vi "FTW-Actor-Initialized.vi"(0 "FTW Actor Instance":refnum<class "FTW-ActorExtended.lvclass">, 5 "Initialized Response":string, 11 "error in":errorcluster) -> (4 "FTW Actor Instance out":refnum<class "FTW-ActorExtended.lvclass">, 15 "error out":errorcluster)   [LabVIEW 2015, in "FTW-ActorExtended.lvclass"]
uses:
  FTW-ActorExtended.lvclass
  FTW-ActorExtended.lvclass/FTW-ActorExtended.ctl
  Instance/FTW-ActorInstance.lvclass
panel:
  out "Initialized Response String":string
  # "Inputs"
  # "Outputs"
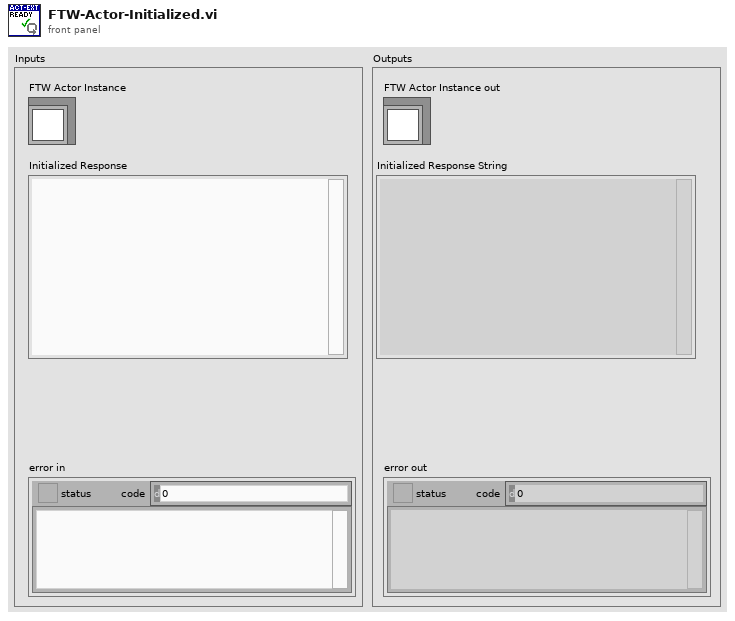
[diagram p1: front panel]
types:
  T1 = typedef "FTW-Type-JSON.ctl" = refnum<data-value>
  T2 = cluster{"Name":string, "URI":string, "Publisher":refnum<class "FTW-Publisher.lvclass">}[]
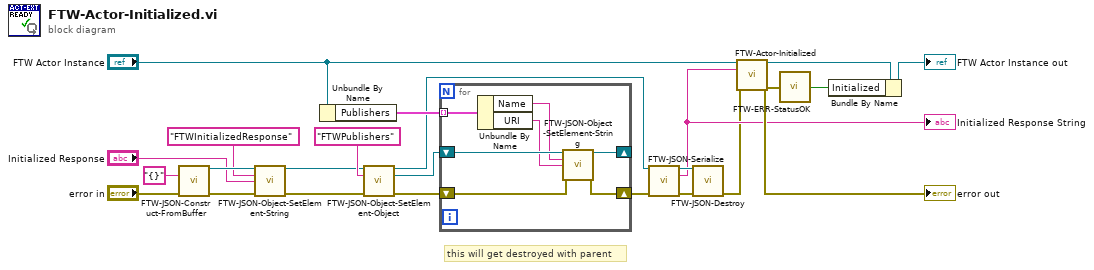
[diagram p0: block diagram]
diagram:
  # "this will get destroyed with parent"
  n1 = call "FTW-JSON-Construct-FromBuffer.vi"("JSON String (UTF-8)"="{}", "error in"="error in") -> ("JSON"=w16:T1, "error out"=w17:errorcluster)  [unwired: 12 in]
  n2 = call "FTW-JSON-Object-SetElement-String.vi"("JSON"=w16, "Key"="FTWInitializedResponse", "Value"="Initialized Response", "error in"=w17) -> ("JSON out"=w3:T1, "error out"=w4:errorcluster)  [unwired: 10 in]
  n3 = Unbundle By Name("FTW Actor Instance") -> ("Publishers"=w12:T2)
  n4 = call "FTW-JSON-Object-SetElement-Object.vi"("JSON Object"=w3, "Key"="FTWPublishers", "error in"=w4) -> ("JSON Root Object"=w7:T1, "JSON Sub-Object"=w10:T1, "error out"=w11:errorcluster)  [unwired: 10 in]
  n5 = for {
    shift-right: [w30] -> w2
    shift-left: w11 -> [w24]
    tunnel: w12 -> [w27] mode=indexing
    shift-right: [w28] -> _
    shift-left: w10 -> [w29]
    n6 = Unbundle By Name(w27) -> ("Name"=w26:string, "URI"=w25:string)
    n7 = call "FTW-JSON-Object-SetElement-String.vi"("JSON"=w29, "Key"=w26, "Value"=w25, "error in"=w24) -> ("JSON out"=w28:T1, "error out"=w30:errorcluster)  [unwired: 10 in]
  }
  n8 = call "FTW-JSON-Serialize.vi"("JSON"=w7, "error in"=w2) -> ("JSON out"=w6:T1, "JSON String (UTF-8)"=w5:string, "error out"=w8:errorcluster)  [unwired: 11 in]
  "Initialized Response String" <- w5
  n9 = call "FTW-JSON-Destroy.vi"("JSON"=w6, "error in"=w8) -> ("error out"=w1:errorcluster)  [unwired: 13 in]
  n10 = call-parent "FTW-Actor-Initialized.vi"("FTW Actor Instance"="FTW Actor Instance", "Initialized Response"=w5, "error in"=w1) -> ("FTW Actor Instance out"=w23:refnum<class "FTW-ActorExtended.lvclass">, "error out"=w21:errorcluster)  [unwired: 11 in]
  "error out" <- w21
  n11 = call "FTW-ERR-StatusOK.vi"("error to check"=w21) -> ("Status OK?"=w20:bool)
  n12 = Bundle By Name(cluster=w23, "Initialized"=w20) -> (→"FTW Actor Instance out":refnum<class "FTW-ActorExtended.lvclass">)
